vi "Write HiddenDevices.vi"(8 "error in (no error)":errorcluster, 10 "HiddenDevices":string[](array[string]), 11 "SetListPrefs in":refnum<class "SetListPrefs.lvclass">) -> (0 "error out":errorcluster, 3 "SetListPrefs out":refnum<class "SetListPrefs.lvclass">)   [LabVIEW 2013, in "SetListPrefs.lvclass"]
uses:
  SetListPrefs.lvclass
  SetListPrefs.lvclass/SetListPrefs.ctl
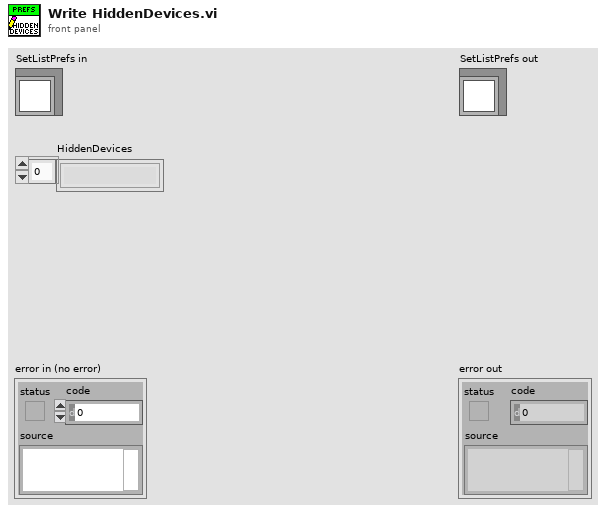
[diagram p1: front panel]
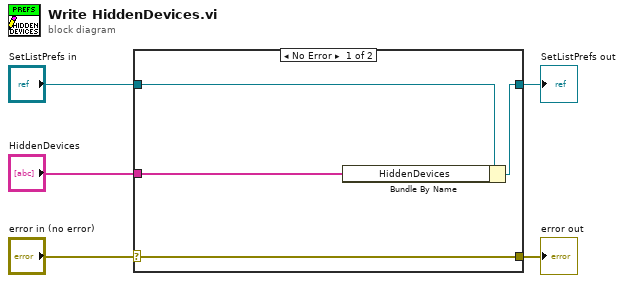
[diagram p0: block diagram]
diagram:
  n1 = case shown="No Error" "error in (no error)" {
    selector: "error in (no error)" -> [w9 w10]
    tunnel: [w9 w10] -> w4
    tunnel: [w7 w11] -> w2
    tunnel: "SetListPrefs in" -> [w8 w11]
    tunnel: "HiddenDevices" -> [w6 _]
    frame No Error {
      n2 = Bundle By Name(cluster=w8, "HiddenDevices"=w6) -> (w7:refnum<class "SetListPrefs.lvclass">)
    }
    frame Error {
    }
  }
  "error out" <- w4
  "SetListPrefs out" <- w2
